vi "dcimgFilenamesToTifStackFilenames.vi"(0 "Base path":path=path "C:/Users/sims01/Desktop/dataAcq", 1 "filenames":string[](array[string])) -> (2 "tifStackFnames":string[](array[string]), 3 "stackFnames":string[](array[string]), 4 "noImgsInStack":dbl)   [LabVIEW 2015]
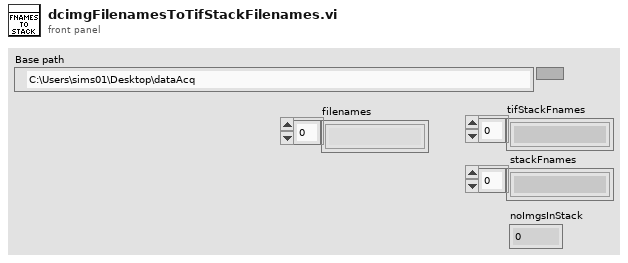
[diagram p1: front panel]
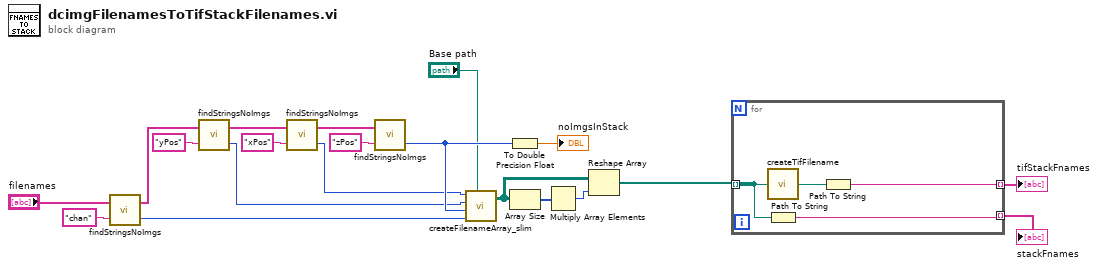
[diagram p0: block diagram]
diagram:
  n1 = call "findStringsNoImgs.vi"("imgProperty"="chan", "filenamesInput"="filenames") -> ("noImgs"=w16:i32, "filenamesOutput"=w13:string[])
  n2 = call "findStringsNoImgs.vi"("imgProperty"="yPos" ("Regular expression"), "filenamesInput"=w13) -> ("noImgs"=w17:i32, "filenamesOutput"=w11:string[])
  n3 = call "findStringsNoImgs.vi"("imgProperty"="xPos" ("Regular expression"), "filenamesInput"=w11) -> ("noImgs"=w18:i32, "filenamesOutput"=w10:string[])
  n4 = call "findStringsNoImgs.vi"("imgProperty"="zPos" ("Regular expression"), "filenamesInput"=w10) -> ("noImgs"=w19:i32)  [unwired: 1 out]
  n5 = call "createFilenameArray_slim.vi"("no x steps"=w18, "no y steps"=w17, "no z steps"=w19, "No colours"=w16, "Base path"="Base path") -> ("stackFnameArray"=w6:path[][][])  [unwired: 1 out]
  n6 = To Double Precision Float(number=w19) -> (double precision float=→"noImgsInStack":dbl)
  n7 = Array Size(array=w6) -> (size(s)=w7:i32[])
  n8 = Multiply Array Elements(1:w7) -> (0:w8:i32)
  n9 = Reshape Array(w6, w8) -> (w5:path[])
  n10 = for {
    tunnel: w5 -> [w24] mode=indexing
    tunnel: [w22] -> w4 mode=indexing
    tunnel: [w21] -> w3 mode=indexing
    n11 = call "createTifFilename.vi"("inputPath"=w24) -> ("tifPath"=w23:path)
    n12 = Path To String(path=w24) -> (string=w21:string)
    n13 = Path To String(path=w23) -> (string=w22:string)
  }
  "tifStackFnames" <- w4
  "stackFnames" <- w3
